vi "Disable Tests.vi"(8 "error in (no error)":errorcluster, 11 "Cluster in":refnum<vi>) -> (0 "error out":errorcluster, 3 "Array":bool[](array[boolean]))   [LabVIEW 2014]
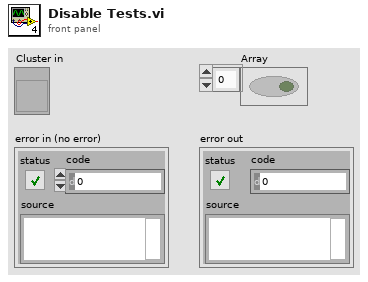
[diagram p1: front panel]
types:
  T1 = enum8{"Enabled", "Disabled", "Disabled and Grayed Out"}
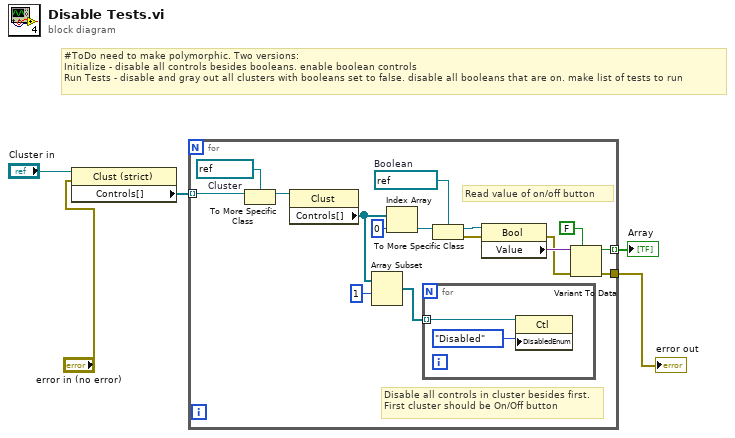
[diagram p0: block diagram]
diagram:
  # "#ToDo need to make polymorphic. Two versions: \nInitialize - disable all controls besides booleans. enable boolean controls\nRun Tests - disable and gray out all clusters with booleans set to false. disable all booleans that are on. make list of tests to run"
  n1 = property class="Clust (strict)"(reference="Cluster in", error in="error in (no error)") -> ("Controls[]"=w2:refnum<vi>[])  [unwired: 2 out]
  n2 = for {
    tunnel: w2 -> [w21] mode=indexing
    tunnel: [w12] -> w3 mode=indexing
    tunnel: [w9] -> w5
    w16 = refnum<vi> refnum  # Boolean
    w19 = refnum<vi> refnum  # Cluster
    # "Read value of on/off button"
    # "Disable all controls in cluster besides first.\nFirst cluster should be On/Off button"
    n3 = To More Specific Class(target class=w19, reference=w21) -> (specific class reference=w20:refnum<vi>)  [unwired: 1 in, 1 out]
    n4 = property class="Clust"(reference=w20) -> ("Controls[]"=w8:refnum<vi>[])  [unwired: 1 in, 2 out]
    n5 = Array Subset(array=w8, index=1) -> (w6:refnum<vi>[])  [unwired: 1 in]
    n6 = Index Array(array=w8, index=0) -> (element=w17:refnum<vi>)
    n7 = for {
      tunnel: w6 -> [w22] mode=indexing
      n8 = property class="Ctl"(reference=w22, "DisabledEnum"=T1."Disabled" ("Disabled")) -> ()  [unwired: 1 in, 2 out]
    }
    n9 = To More Specific Class(target class=w16, reference=w17) -> (specific class reference=w11:refnum<vi>, error out=w15:errorcluster)  [unwired: 1 in]
    n10 = property class="Bool"(reference=w11, error in=w15) -> (error out=w10:errorcluster, "Value"=w14:variant)  [unwired: 1 out]
    n11 = Variant To Data(error in=w10, type=FALSE, Variant=w14) -> (data=w12:bool, error out=w9:errorcluster)
  }
  "error out" <- w5
  "Array" <- w3
